vi "unicodeStringToASCII.vi"(8 "error in (no error)":errorcluster, 10 "Unicode String":string) -> (0 "error out":errorcluster, 2 "ASCII String":string)   [LabVIEW 2017, in "JKI Simple Localization.lvlib"]
uses:
  API/JKI Simple Localization.lvlib
  kernel32.dll
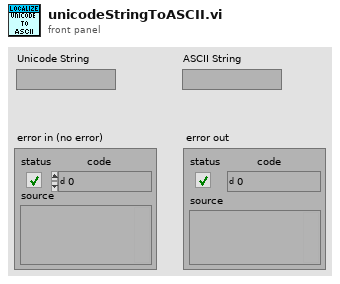
[diagram p1: front panel]
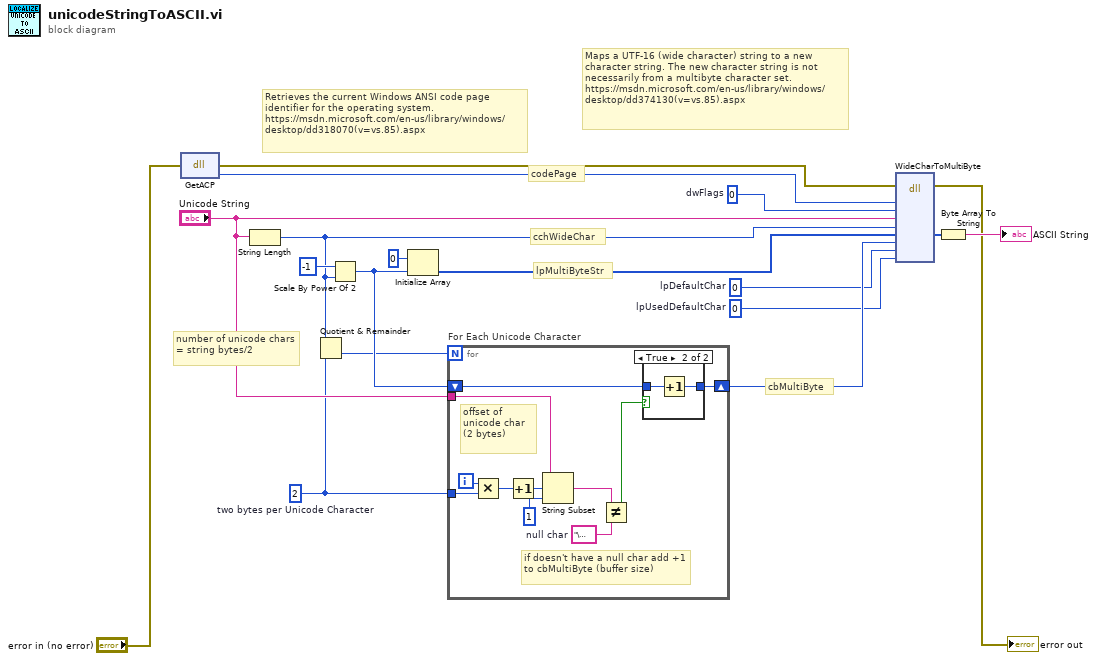
[diagram p0: block diagram]
diagram:
  w4 = u32 0  # lpDefaultChar
  w5 = u32 0  # lpUsedDefaultChar
  w6 = 2  # two bytes per Unicode Character
  w16 = u32 0  # dwFlags
  # "Retrieves the current Windows ANSI code page identifier for the operating system.\nhttps://msdn.microsoft.com/en-us/library/windows/desktop/dd318070(v=vs.85).aspx"
  # "codePage"
  # "Maps a UTF-16 (wide character) string to a new character string. The new character string is not necessarily from a multibyte character set.\nhttps://msdn.microsoft.com/en-us/library/windows/desktop/dd374130(v=vs.85).aspx"
  # "cchWideChar"
  # "lpMultiByteStr"
  # "cbMultiByte"
  # "number of unicode chars = string bytes/2"
  n1 = dll-call lib="kernel32.dll" fn="GetACP" label="kernel32.dll\nGetACP"(error in="error in (no error)") -> (error out=w3:errorcluster, w18:u32)  [unwired: 2 in, 1 out]
  n2 = String Length(string="Unicode String") -> (length=w10:i32)
  n3 = Quotient & Remainder(x=w10, y=w6) -> (floor(x/y)=w7:i32)  [unwired: 1 out]
  n4 = Scale By Power Of 2(n=-1, x=w10) -> (x*2^n=w9:i32)
  n5 = Initialize Array(u8 0, w9) -> (w17:u8[])
  n6 = for "For Each Unicode Character" {
    N: w7 -> [_]
    tunnel: w6 -> [w28]
    tunnel: "Unicode String" -> [w26]
    shift-right: [w19] -> w8
    shift-left: w9 -> [w20]
    i -> [w29]
    w22 = "\u0000"  # null char
    # "if doesn't have a null char add +1 to cbMultiByte (buffer size)"
    # "offset of unicode char (2 bytes)"
    n7 = Multiply(x=w29, y=w28) -> (x*y=w27:i32)
    n8 = Increment(x=w27) -> (x+1=w24:i32)
    n9 = String Subset(string=w26, offset (0)=w24, length (rest)=1 ("length (rest)")) -> (substring=w23:string)
    n10 = Not Equal?(x=w23, y=w22) -> (x != y?=w21:bool)
    n11 = case shown="True" w21 {
      tunnel: w20 -> [w30 w32]
      tunnel: [w30 w31] -> w19
      frame False {
      }
      frame True {
        n12 = Increment(x=w32) -> (x+1=w31:i32)
      }
    }
  }
  n13 = dll-call lib="kernel32.dll" fn="WideCharToMultiByte" label="kernel32.dll\nWideCharToMultiByte"(error in=w3, "codePage"=w18, "dwFlags"=w16, "lpWideCharStr"="Unicode String", "cchWideChar"=w10, "lpMultiByteStr"=w17, "cbMultiByte"=w8, "lpDefaultChar"=w4, "lpUsedDefaultChar"=w5) -> (error out=→"error out":errorcluster, "lpMultiByteStr"=w13:u8[])  [unwired: 9 in, 2 out]
  n14 = Byte Array To String(unsigned byte array=w13) -> (string=→"ASCII String":string)
